vi "ErrCheck_Valid Params Number.vi"(8 "Error In":errorcluster, 11 "Macro Command String IN":string="LOOP.Start\t(loop.iterations,3.000);") -> (0 "Error Out":errorcluster, 2 "Less params than expected?":bool, 3 "More params than expected?":bool)   [LabVIEW 2012]
doc: "SciScan 1.2 160622"
uses:
  <vilib>/Utility/error.llb/whitespace.ctl
  MacroRules_FGV_Commands.ctl
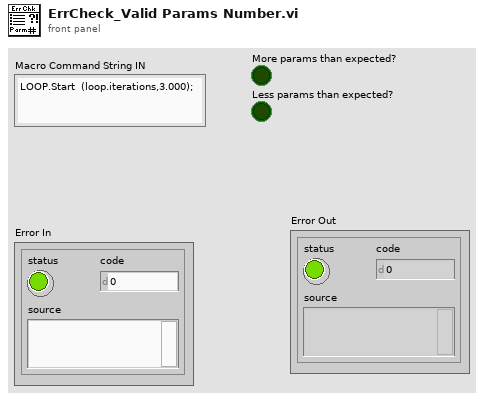
[diagram p1: front panel]
types:
  T1 = typedef "MacroRules_FGV_Commands.ctl" = enum16{"Read File", "Get All", "Get Param and Flags"}
  T2 = typedef "whitespace.ctl" = u16
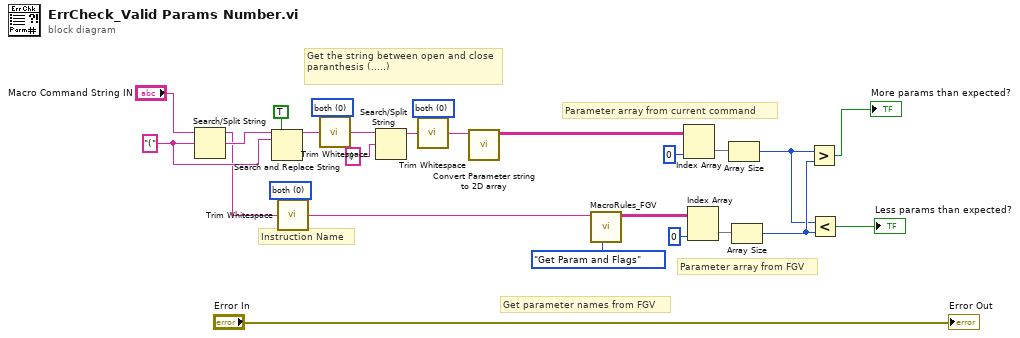
[diagram p0: block diagram]
diagram:
  w14 = T2 0 items=["both", "start of string", "end of string"] ("location (both)")
  w23 = T2 0 items=["both", "start of string", "end of string"] ("location (both)")
  w26 = T2 0 items=["both", "start of string", "end of string"] ("location (both)")
  w18 = "(" ("search string/char (-)")
  # "Parameter array from current command"
  # "Parameter array from FGV"
  # "Get parameter names from FGV"
  # "Instruction Name"
  # "Get the string between open and close paranthesis (.....)"
  n1 = Search/Split String(string="Macro Command String IN", search string/char (-)=w18) -> (substring before match=w13:string, match + rest of string=w17:string)  [unwired: 1 in, 1 out]
  n2 = Search and Replace String(replace all?=TRUE ("replace all? (F)"), input string=w17, search string=w18) -> (result string=w19:string)  [unwired: 5 in, 3 out]
  n3 = call <vilib>:"Trim Whitespace.vi"("string"=w13, "location (both)"=w14) -> ("trimmed string"=w1:string)
  n4 = call <vilib>:"Trim Whitespace.vi"("string"=w19, "location (both)"=w26) -> ("trimmed string"=w16:string)
  n5 = Search/Split String(string=w16, search string/char (-)=")") -> (substring before match=w24:string)  [unwired: 1 in, 2 out]
  n6 = call <vilib>:"Trim Whitespace.vi"("string"=w24, "location (both)"=w23) -> ("trimmed string"=w15:string)
  n7 = call "Convert Parameter string to 2D array.vi"("Parameter string IN (without paranthesis)"=w15) -> ("Params table OUT"=w2:string[][])  [unwired: 7 in, 3 out]
  n8 = call "MacroRules_FGV.vi"("MacroRules_FGV_Commands"=MacroRules_FGV_Commands."Get Param and Flags", "Command Name IN"=w1) -> ("Parameters"=w3:string[][])  [unwired: 5 in, 4 out]
  n9 = Index Array(array=w2, index (col)=0 ("disabled index (col)")) -> (element=w9:string[])  [unwired: 1 in]
  n10 = Index Array(array=w3, index (col)=0 ("disabled index (col)")) -> (element=w11:string[])  [unwired: 1 in]
  n11 = Array Size(array=w9) -> (size(s)=w4:i32)
  n12 = Array Size(array=w11) -> (size(s)=w5:i32)
  n13 = Greater?(x=w4, y=w5) -> (0:→"More params than expected?":bool)
  n14 = Less?(x=w4, y=w5) -> (x < y?=→"Less params than expected?":bool)
  "Error Out" <- "Error In"
